vi "OpenCL Test.vi"() -> ()   [LabVIEW 2012]
uses:
  OpenCL States.ctl
  <vilib>/RaptorView/OpenCLV/User Controls/Array Dimensions.ctl
panel:
  out "Compute":u32
  out "Write":u32
  out "Read":u32
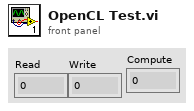
[diagram p1: front panel]
types:
  T1 = typedef "OpenCL States.ctl" = enum16{"Allocate Memory", "Compile Kernels", "Create Device", "Write", "Read", "Operate", "Delete Memory", "Delete"}
  T2 = typedef "Array Dimensions.ctl" = cluster{"Depth":u64, "Height":u64, "Width":u64}
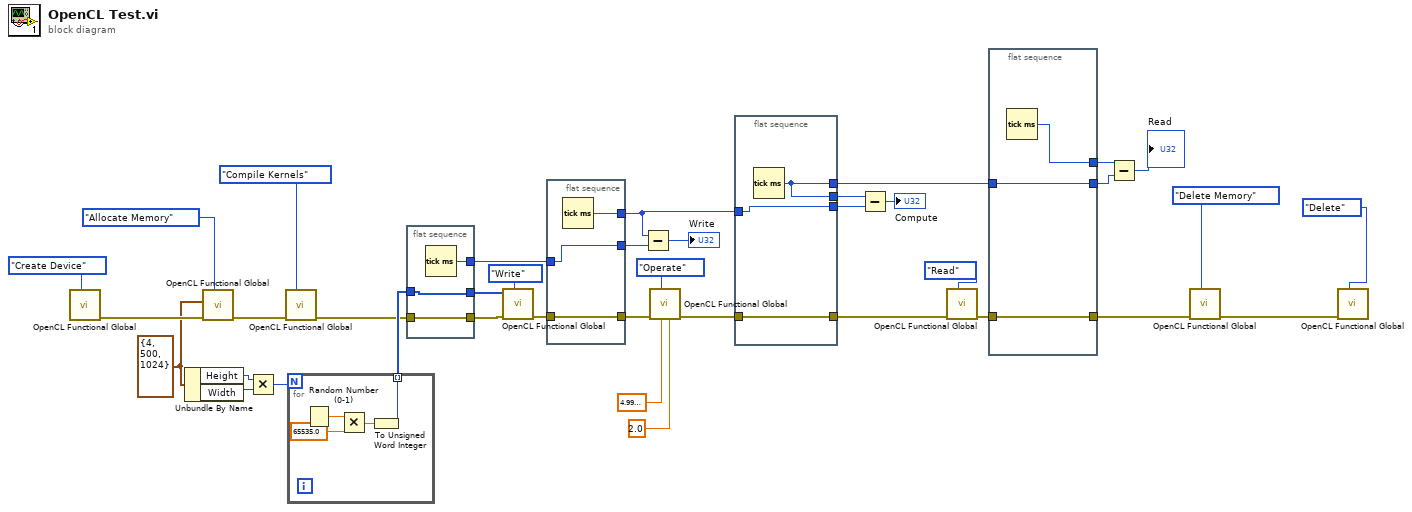
[diagram p0: block diagram]
diagram:
  w21 = T2 {"Depth"=4, "Height"=500, "Width"=1024} ("Dimension")
  n1 = call "OpenCL Functional Global.vi"("States"=OpenCL_States."Create Device") -> ("Error Out"=w37:errorcluster)  [unwired: 8 in, 2 out]
  n2 = Unbundle By Name(w21) -> ("Height"=w33:u64, "Width"=w32:u64)
  n3 = call "OpenCL Functional Global.vi"("States"=OpenCL_States."Allocate Memory", "Error In"=w37, "Dimension"=w21) -> ("Error Out"=w35:errorcluster)  [unwired: 6 in, 2 out]
  n4 = Multiply(x=w33, y=w32) -> (x*y=w31:u64)
  n5 = call "OpenCL Functional Global.vi"("States"=OpenCL_States."Compile Kernels", "Error In"=w35) -> ("Error Out"=w1:errorcluster)  [unwired: 7 in, 2 out]
  n6 = for {
    N: w31 -> [_]
    tunnel: [w39] -> w3 mode=indexing
    n7 = Random Number (0-1)() -> (number: 0 to 1=w42:dbl)
    n8 = Multiply(x=w42, y=65535.0) -> (x*y=w40:dbl)
    n9 = To Unsigned Word Integer(number=w40) -> (unsigned 16bit integer=w39:u16)
  }
  n10 = flat-sequence {
    tunnel: [w44] -> w29
    tunnel: [w45] -> w16
    tunnel: w3 -> [w44]
    tunnel: [w43] -> w2
    tunnel: w1 -> [w43]
    frame #0 {
      n11 = Tick Count (ms)() -> (millisecond timer value=w45:u32)
    }
  }
  n12 = call "OpenCL Functional Global.vi"("States"=OpenCL_States."Write", "Error In"=w2, "B-Scan"=w29) -> ("Error Out"=w17:errorcluster)  [unwired: 6 in, 2 out]
  n13 = flat-sequence {
    tunnel: [w48] -> w18
    tunnel: w17 -> [w48]
    tunnel: w16 -> [w47]
    tunnel: [w47] -> w15
    tunnel: [w46] -> w11
    frame #0 {
      n14 = Tick Count (ms)() -> (millisecond timer value=w46:u32)
    }
  }
  n15 = Subtract(x=w11, y=w15) -> (x-y=→"Write":u32)
  n16 = call "OpenCL Functional Global.vi"("Gain"=sgl 2.0 ("Bias"), "Bias"=sgl 5e-05, "States"=OpenCL_States."Operate", "Error In"=w18) -> ("Error Out"=w13:errorcluster)  [unwired: 5 in, 2 out]
  n17 = flat-sequence {
    tunnel: [w51] -> w14
    tunnel: w13 -> [w51]
    tunnel: w11 -> [w50]
    tunnel: [w50] -> w10
    tunnel: [w49] -> w9
    tunnel: [w49] -> w7
    frame #0 {
      n18 = Tick Count (ms)() -> (millisecond timer value=w49:u32)
    }
  }
  n19 = Subtract(x=w9, y=w10) -> (x-y=→"Compute":u32)
  n20 = call "OpenCL Functional Global.vi"("States"=OpenCL_States."Read", "Error In"=w14) -> ("Error Out"=w20:errorcluster)  [unwired: 7 in, 2 out]
  n21 = flat-sequence {
    tunnel: w20 -> [w54]
    tunnel: [w54] -> w19
    tunnel: [w53] -> w6
    tunnel: w7 -> [w52]
    tunnel: [w52] -> w5
    frame #0 {
      n22 = Tick Count (ms)() -> (millisecond timer value=w53:u32)
    }
  }
  n23 = Subtract(x=w6, y=w5) -> (x-y=→"Read":u32)
  n24 = call "OpenCL Functional Global.vi"("States"=OpenCL_States."Delete Memory", "Error In"=w19) -> ("Error Out"=w25:errorcluster)  [unwired: 7 in, 2 out]
  n25 = call "OpenCL Functional Global.vi"("States"=OpenCL_States."Delete", "Error In"=w25) -> ()  [unwired: 7 in, 3 out]
